vi "Process CAN Frame.vi"(10 "CAN frame":T1 {"type" items=["CAN Data", "CAN Remote"]; "identifier" format="%.0x"}) -> ()   [LabVIEW 2014]
uses:
  <vilib>/RioEmbeddedCAN/RioEmbeddedCAN.llb/CANFrameControl.ctl
  MC/MC Temp 1.ctl
  MC/MC Temp 2.ctl
  MC/MC Temp 3.ctl
  MC/MC Position.ctl
  MC/MC Current.ctl
  MC/MC Voltage.ctl
  MC/MC State.ctl
  Inverter States.ctl
  Inverter Run Modes.ctl
  VSM States.ctl
  MC/MC Faults.ctl
  MC/MC Post Faults.ctl
  MC/MC Run Faults.ctl
  MC/MC Torque.ctl
  Global Data.vi
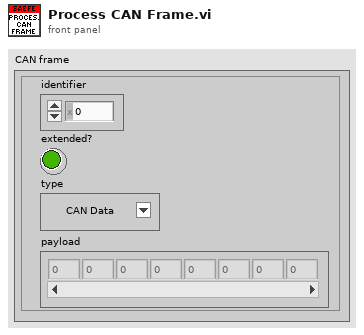
[diagram p1: front panel]
types:
  T1 = typedef "CANFrameControl.ctl" = cluster{"identifier":u32, "extended?":bool, "type":u8, "payload":u8[]}
  T2 = typedef "MC Temp 1.ctl" = cluster{"IGBT A (C)":dbl, "IGBT B (C)":dbl, "IGBT C (C)":dbl, "Gate Driver (C)":dbl}
  T3 = typedef "MC Temp 2.ctl" = cluster{"Control Board (C)":dbl, "RTD #1":dbl, "RTD #2":dbl, "RTD #3":dbl}
  T4 = typedef "MC Temp 3.ctl" = cluster{"RTD #4":dbl, "RTD #5":dbl, "Motor (C)":dbl, "T-Shudder":dbl}
  T5 = typedef "MC Position.ctl" = cluster{"Motor Angle":dbl, "Motor Speed":dbl, "Electrical Output Freq.":dbl, "Delta Resolver Filt.":dbl}
  T6 = typedef "MC Current.ctl" = cluster{"I-Phase A":dbl, "I-Phase B":dbl, "I-Phase C":dbl, "I-Battery":dbl}
  T7 = typedef "MC Voltage.ctl" = cluster{"V-Phase AB":dbl, "V-Phase BC":dbl, "V-Output":dbl, "V-Battery":dbl}
  T8 = typedef "MC State.ctl" = cluster{"Inverter":T9, "Inv. Run Mode":T10, "Inv. Command":enum16{"CAN Mode", "VSM Mode"}, "Inv. Enable":enum16{"Inverter Disabled", "Inverter Enabled"}, "Inv. Enable Lock":enum16{"Inverter Locked", "Inverter Unlocked"}, "Direction":enum16{"Forward", "Reverse/Stopped"}, "VSM States":T11, "Relay 1":bool, "Relay 2":bool, "Relay 3":bool, "Relay 4":bool}
  T9 = typedef "Inverter States.ctl" = enum16{"Power On", "Stop", "Open Loop", "Closed Loop", "Wait", "Internal", "Idle Run", "Idle Stop", ""}
  T10 = typedef "Inverter Run Modes.ctl" = enum16{"Torque Mode", "Speed Mode"}
  T11 = typedef "VSM States.ctl" = enum16{"VSM Start", "Pre-Charge Init", "Pre-Charge Active", "Pre-Charge Complete", "VSM Wait", "VSM Ready", "Motor Running", "Blink Fault Code", "Shutdown in Process", "Recycle Power"}
  T12 = typedef "MC Faults.ctl" = cluster{"POST":T13, "RUN":T14}
  T13 = typedef "MC Post Faults.ctl" = enum32{"None"}
  T14 = typedef "MC Run Faults.ctl" = enum32{"None"}
  T15 = typedef "MC Torque.ctl" = cluster{"T-Requested (Telem)":dbl, "T-Feedback":dbl}
  T16 = enum16{"Off", "On, Not Charging", "Charging", "Charging Finished", "Charging Error"}
  T17 = enum16{"Disconnected", "Pre-charging", "Main Charging", "Balancing", "Charging Finished OK", "Charging Error"}
  T18 = typedef "BMS Telemetry.ctl" = cluster{"Ignition":bool, "Charger Mains":bool, "Fast Charge":bool, "Simple Charger Enabled":bool, "Car State":enum16{"Off", "On, Not Charging", "Charging", "Charging Finished", "Charging Error"}, "Charging State":enum16{"Disconnected", "Pre-charging", "Main Charging", "Balancing", "Charging Finished OK", "Charging Error"}, "Charging Stage Duration":u16, "Last Charging Error":enum16{"No Error", "Cell Voltage Too Low", "No Comm from Cells so can't start", "Maximum charging stage duration expired", "No Comm from Cels so can't balande", "Cannot set balancing voltage", "Cell temps too high", "No Comms so can't determine temp", "# of Cells Mismatch", "Cells Overvoltage", "Cell Protection Event occured."}, "Number of Detected Cells":u8, "Under-Voltage":bool, "Over-Voltage":bool, "Overheat":bool, "Leakage":bool, "No Cell Comms":bool, "Low Voltage":bool, "High Temperature":bool, "Min Cell V":dbl, "Max Cell V":dbl, "Mean Cell V":dbl, "Total V":dbl, "Min Cell t":dbl, "Max Cell t":dbl, "Mean Cell t":dbl, "Cell Voltages":cluster{"[0]":dbl, "[1]":dbl, "[2]":dbl, "[3]":dbl, "[4]":dbl, "[5]":dbl, "[6]":dbl, "[7]":dbl, "[8]":dbl, "[9]":dbl, "[10]":dbl, "[11]":dbl, "[12]":dbl, "[13]":dbl, "[14]":dbl, "[15]":dbl, "[16]":dbl, "[17]":dbl, "[18]":dbl, "[19]":dbl, "[20]":dbl, "[21]":dbl, "[22]":dbl, "[23]":dbl, "[24]":dbl, "[25]":dbl, "[26]":dbl, "[27]":dbl, "[28]":dbl, "[29]":dbl, "[30]":dbl, "[31]":dbl, "[32]":dbl, "[33]":dbl, "[34]":dbl, "[35]":dbl, "[36]":dbl, "[37]":dbl, "[38]":dbl, "[39]":dbl, "[40]":dbl, "[41]":dbl, "[42]":dbl, "[43]":dbl, "[44]":dbl, "[45]":dbl, "[46]":dbl, "[47]":dbl, "[48]":dbl, "[49]":dbl, "[50]":dbl, "[51]":dbl, "[52]":dbl, "[53]":dbl, "[54]":dbl, "[55]":dbl, "[56]":dbl, "[57]":dbl, "[58]":dbl, "[59]":dbl, "[60]":dbl, "[61]":dbl, "[62]":dbl, "[63]":dbl, "[64]":dbl, "[65]":dbl, "[66]":dbl, "[67]":dbl, "[68]":dbl, "[69]":dbl, "[70]":dbl}, "Cell Temps":cluster{"[0]":dbl, "[1]":dbl, "[2]":dbl, "[3]":dbl, "[4]":dbl, "[5]":dbl, "[6]":dbl, "[7]":dbl, "[8]":dbl, "[9]":dbl, "[10]":dbl, "[11]":dbl, "[12]":dbl, "[13]":dbl, "[14]":dbl, "[15]":dbl, "[16]":dbl, "[17]":dbl, "[18]":dbl, "[19]":dbl, "[20]":dbl, "[21]":dbl, "[22]":dbl, "[23]":dbl, "[24]":dbl, "[25]":dbl, "[26]":dbl, "[27]":dbl, "[28]":dbl, "[29]":dbl, "[30]":dbl, "[31]":dbl, "[32]":dbl, "[33]":dbl, "[34]":dbl, "[35]":dbl, "[36]":dbl, "[37]":dbl, "[38]":dbl, "[39]":dbl, "[40]":dbl, "[41]":dbl, "[42]":dbl, "[43]":dbl, "[44]":dbl, "[45]":dbl, "[46]":dbl, "[47]":dbl, "[48]":dbl, "[49]":dbl, "[50]":dbl, "[51]":dbl, "[52]":dbl, "[53]":dbl, "[54]":dbl, "[55]":dbl, "[56]":dbl, "[57]":dbl, "[58]":dbl, "[59]":dbl, "[60]":dbl, "[61]":dbl, "[62]":dbl, "[63]":dbl, "[64]":dbl, "[65]":dbl, "[66]":dbl, "[67]":dbl, "[68]":dbl, "[69]":dbl, "[70]":dbl}}
  T19 = cluster{"[0]":dbl, "[1]":dbl, "[2]":dbl, "[3]":dbl, "[4]":dbl, "[5]":dbl, "[6]":dbl, "[7]":dbl, "[8]":dbl, "[9]":dbl, "[10]":dbl, "[11]":dbl, "[12]":dbl, "[13]":dbl, "[14]":dbl, "[15]":dbl, "[16]":dbl, "[17]":dbl, "[18]":dbl, "[19]":dbl, "[20]":dbl, "[21]":dbl, "[22]":dbl, "[23]":dbl, "[24]":dbl, "[25]":dbl, "[26]":dbl, "[27]":dbl, "[28]":dbl, "[29]":dbl, "[30]":dbl, "[31]":dbl, "[32]":dbl, "[33]":dbl, "[34]":dbl, "[35]":dbl, "[36]":dbl, "[37]":dbl, "[38]":dbl, "[39]":dbl, "[40]":dbl, "[41]":dbl, "[42]":dbl, "[43]":dbl, "[44]":dbl, "[45]":dbl, "[46]":dbl, "[47]":dbl, "[48]":dbl, "[49]":dbl, "[50]":dbl, "[51]":dbl, "[52]":dbl, "[53]":dbl, "[54]":dbl, "[55]":dbl, "[56]":dbl, "[57]":dbl, "[58]":dbl, "[59]":dbl, "[60]":dbl, "[61]":dbl, "[62]":dbl, "[63]":dbl, "[64]":dbl, "[65]":dbl, "[66]":dbl, "[67]":dbl, "[68]":dbl, "[69]":dbl, "[70]":dbl}
  T20 = cluster{"Cell Voltages[0]":dbl, "Cell Voltages[1]":dbl, "Cell Voltages[2]":dbl, "Cell Voltages[3]":dbl, "Cell Voltages[4]":dbl, "Cell Voltages[5]":dbl, "Cell Voltages[6]":dbl, "Cell Voltages[7]":dbl, "Cell Voltages[8]":dbl, "Cell Voltages[9]":dbl, "Cell Voltages[10]":dbl, "Cell Voltages[11]":dbl, "Cell Voltages[12]":dbl, "Cell Voltages[13]":dbl, "Cell Voltages[14]":dbl, "Cell Voltages[15]":dbl, "Cell Voltages[16]":dbl, "Cell Voltages[17]":dbl, "Cell Voltages[18]":dbl, "Cell Voltages[19]":dbl, "Cell Voltages[20]":dbl, "Cell Voltages[21]":dbl, "Cell Voltages[22]":dbl, "Cell Voltages[23]":dbl, "Cell Voltages[24]":dbl, "Cell Voltages[25]":dbl, "Cell Voltages[26]":dbl, "Cell Voltages[27]":dbl, "Cell Voltages[28]":dbl, "Cell Voltages[29]":dbl, "Cell Voltages[30]":dbl, "Cell Voltages[31]":dbl, "Cell Voltages[32]":dbl, "Cell Voltages[33]":dbl, "Cell Voltages[34]":dbl, "Cell Voltages[35]":dbl, "Cell Voltages[36]":dbl, "Cell Voltages[37]":dbl, "Cell Voltages[38]":dbl, "Cell Voltages[39]":dbl, "Cell Voltages[40]":dbl, "Cell Voltages[41]":dbl, "Cell Voltages[42]":dbl, "Cell Voltages[43]":dbl, "Cell Voltages[44]":dbl, "Cell Voltages[45]":dbl, "Cell Voltages[46]":dbl, "Cell Voltages[47]":dbl, "Cell Voltages[48]":dbl, "Cell Voltages[49]":dbl, "Cell Voltages[50]":dbl, "Cell Voltages[51]":dbl, "Cell Voltages[52]":dbl, "Cell Voltages[53]":dbl, "Cell Voltages[54]":dbl, "Cell Voltages[55]":dbl, "Cell Voltages[56]":dbl, "Cell Voltages[57]":dbl, "Cell Voltages[58]":dbl, "Cell Voltages[59]":dbl, "Cell Voltages[60]":dbl, "Cell Voltages[61]":dbl, "Cell Voltages[62]":dbl, "Cell Voltages[63]":dbl, "Cell Voltages[64]":dbl, "Cell Voltages[65]":dbl, "Cell Voltages[66]":dbl, "Cell Voltages[67]":dbl, "Cell Voltages[68]":dbl, "Cell Voltages[69]":dbl, "Cell Voltages[70]":dbl}
  T21 = cluster{"Cell Temps[0]":dbl, "Cell Temps[1]":dbl, "Cell Temps[2]":dbl, "Cell Temps[3]":dbl, "Cell Temps[4]":dbl, "Cell Temps[5]":dbl, "Cell Temps[6]":dbl, "Cell Temps[7]":dbl, "Cell Temps[8]":dbl, "Cell Temps[9]":dbl, "Cell Temps[10]":dbl, "Cell Temps[11]":dbl, "Cell Temps[12]":dbl, "Cell Temps[13]":dbl, "Cell Temps[14]":dbl, "Cell Temps[15]":dbl, "Cell Temps[16]":dbl, "Cell Temps[17]":dbl, "Cell Temps[18]":dbl, "Cell Temps[19]":dbl, "Cell Temps[20]":dbl, "Cell Temps[21]":dbl, "Cell Temps[22]":dbl, "Cell Temps[23]":dbl, "Cell Temps[24]":dbl, "Cell Temps[25]":dbl, "Cell Temps[26]":dbl, "Cell Temps[27]":dbl, "Cell Temps[28]":dbl, "Cell Temps[29]":dbl, "Cell Temps[30]":dbl, "Cell Temps[31]":dbl, "Cell Temps[32]":dbl, "Cell Temps[33]":dbl, "Cell Temps[34]":dbl, "Cell Temps[35]":dbl, "Cell Temps[36]":dbl, "Cell Temps[37]":dbl, "Cell Temps[38]":dbl, "Cell Temps[39]":dbl, "Cell Temps[40]":dbl, "Cell Temps[41]":dbl, "Cell Temps[42]":dbl, "Cell Temps[43]":dbl, "Cell Temps[44]":dbl, "Cell Temps[45]":dbl, "Cell Temps[46]":dbl, "Cell Temps[47]":dbl, "Cell Temps[48]":dbl, "Cell Temps[49]":dbl, "Cell Temps[50]":dbl, "Cell Temps[51]":dbl, "Cell Temps[52]":dbl, "Cell Temps[53]":dbl, "Cell Temps[54]":dbl, "Cell Temps[55]":dbl, "Cell Temps[56]":dbl, "Cell Temps[57]":dbl, "Cell Temps[58]":dbl, "Cell Temps[59]":dbl, "Cell Temps[60]":dbl, "Cell Temps[61]":dbl, "Cell Temps[62]":dbl, "Cell Temps[63]":dbl, "Cell Temps[64]":dbl, "Cell Temps[65]":dbl, "Cell Temps[66]":dbl, "Cell Temps[67]":dbl, "Cell Temps[68]":dbl, "Cell Temps[69]":dbl, "Cell Temps[70]":dbl}
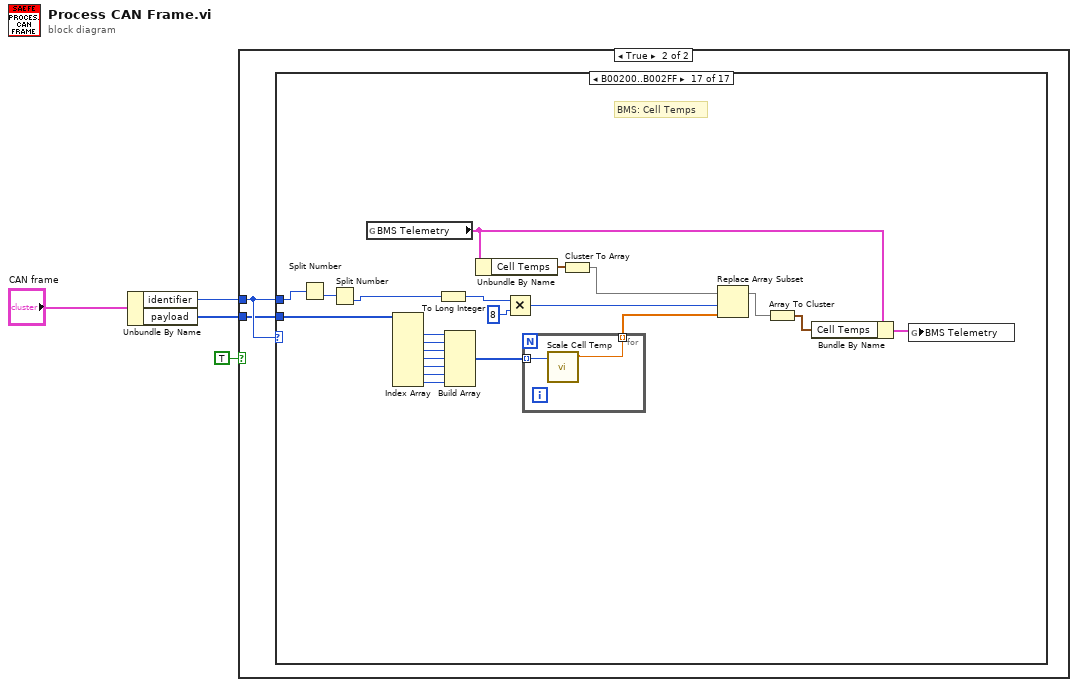
[diagram p0: block diagram]
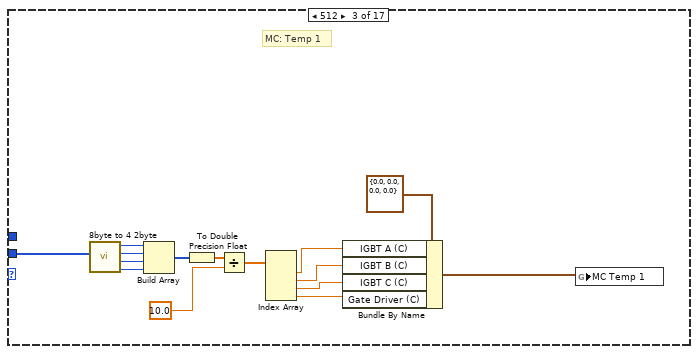
[diagram p5: hidden frame]
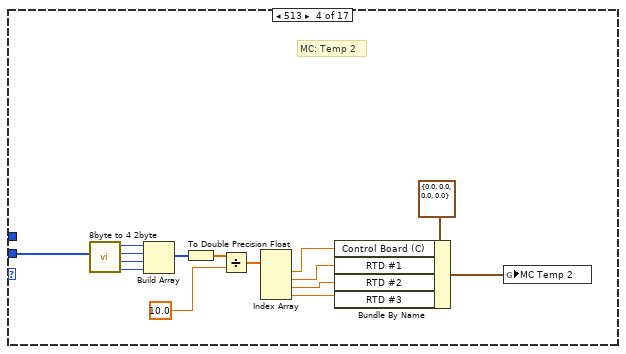
[diagram p6: hidden frame]
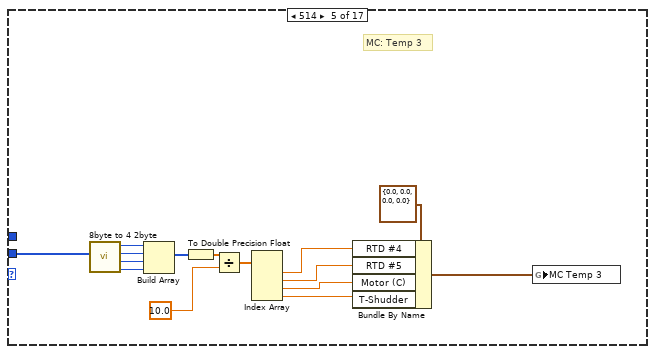
[diagram p7: hidden frame]
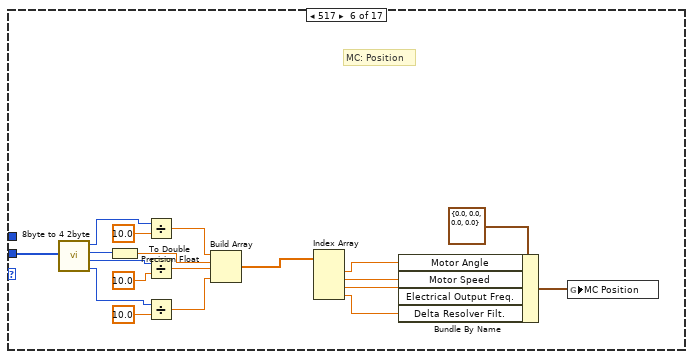
[diagram p8: hidden frame]
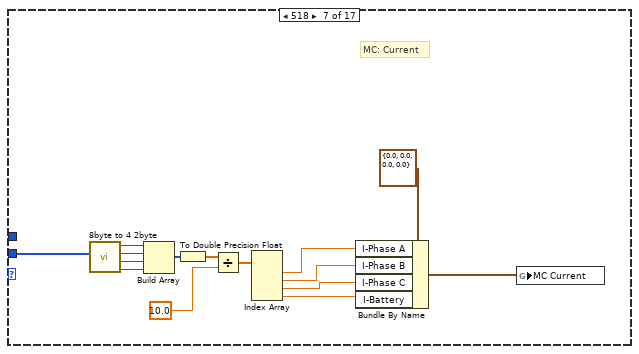
[diagram p9: hidden frame]
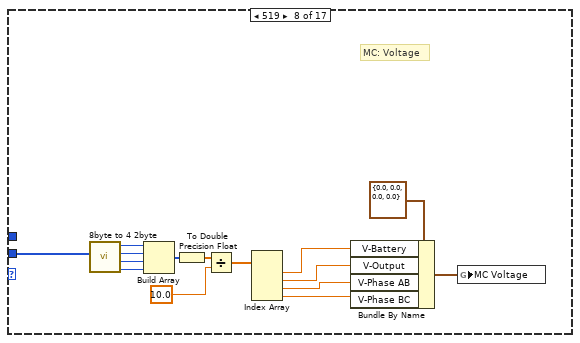
[diagram p10: hidden frame]
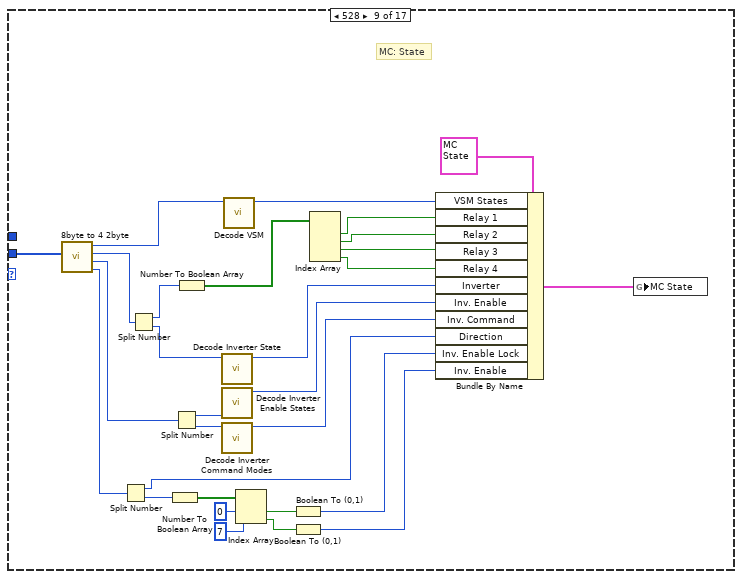
[diagram p11: hidden frame]
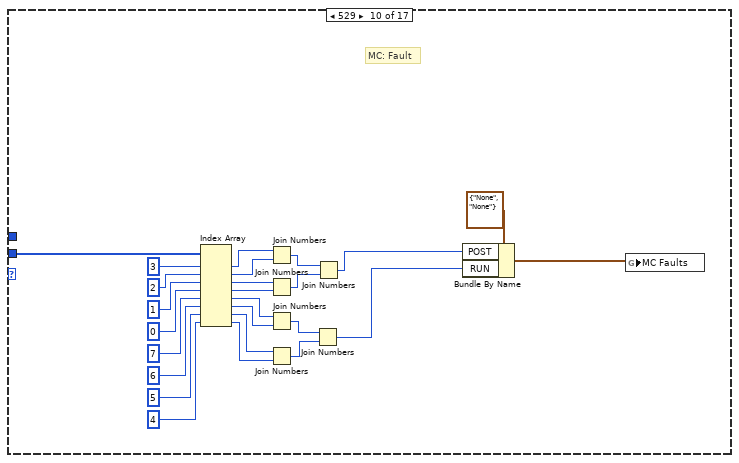
[diagram p12: hidden frame]
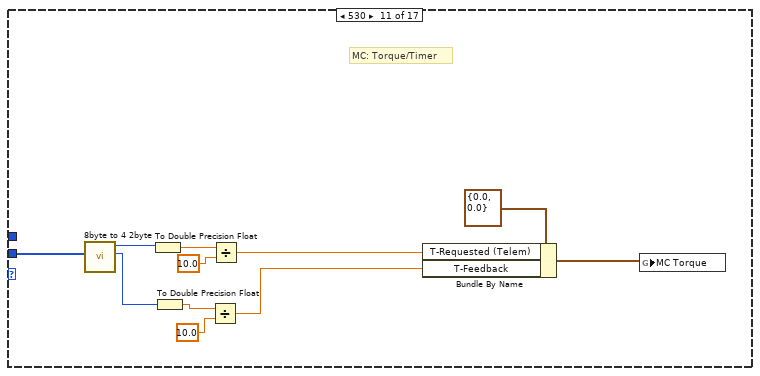
[diagram p13: hidden frame]
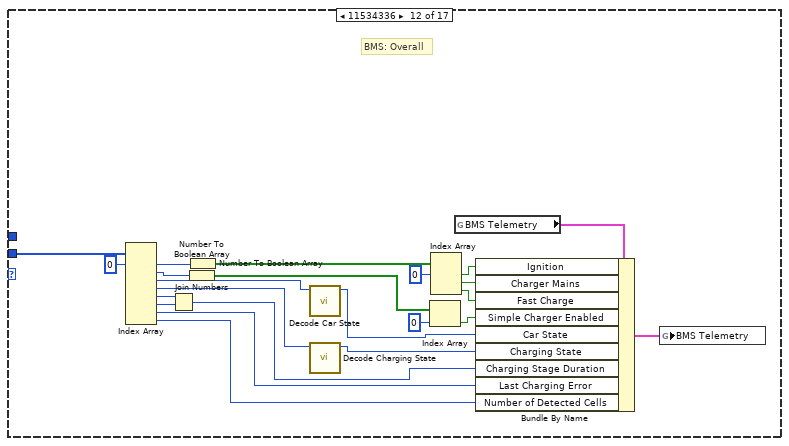
[diagram p14: hidden frame]
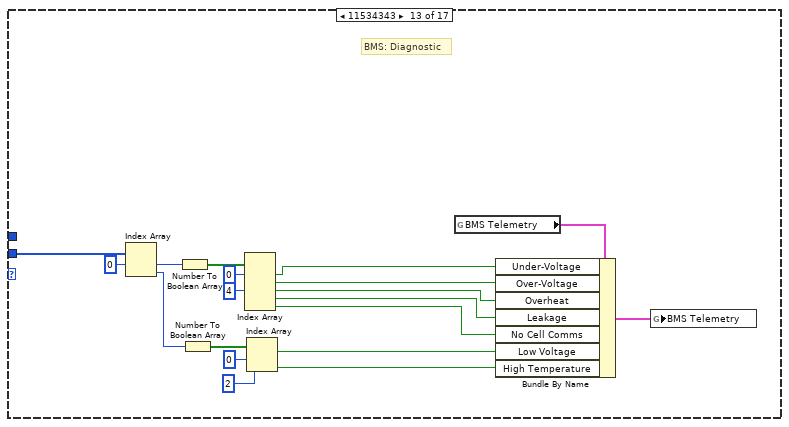
[diagram p15: hidden frame]
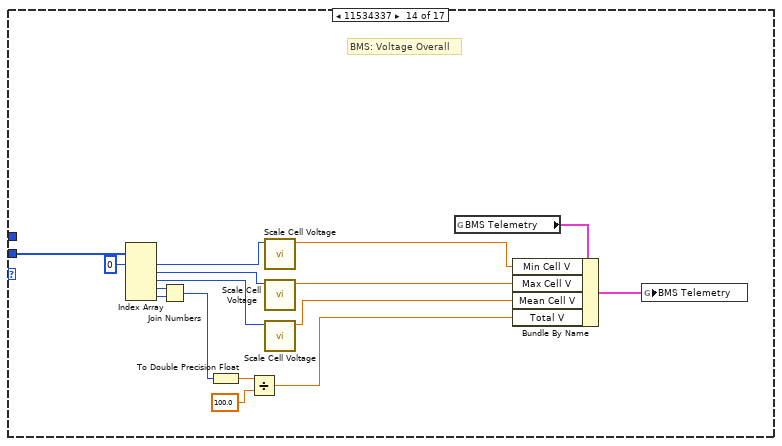
[diagram p16: hidden frame]
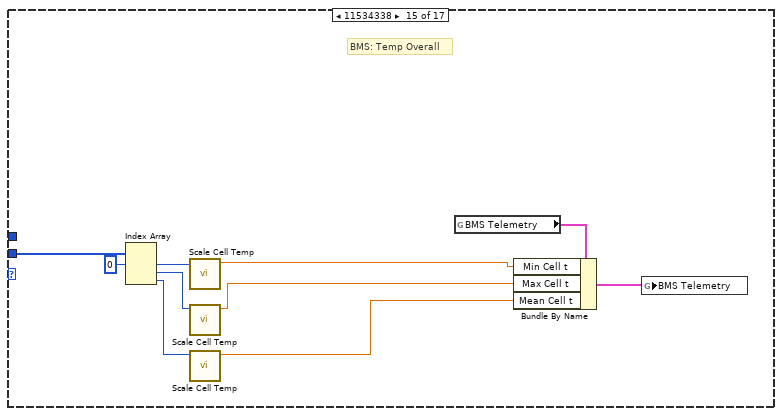
[diagram p17: hidden frame]
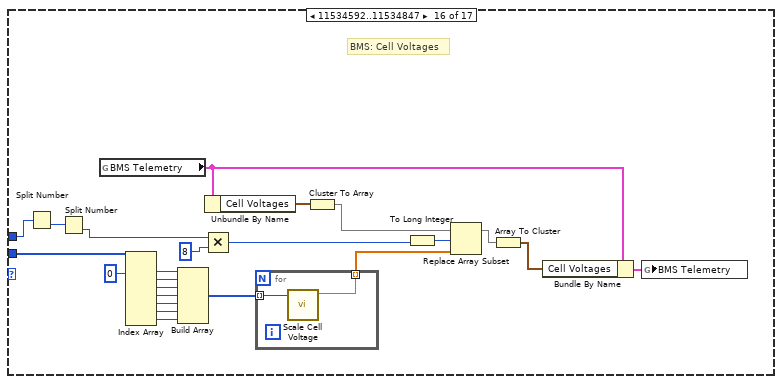
[diagram p18: hidden frame]
diagram:
  n1 = Unbundle By Name("CAN frame") -> ("identifier"=w3:u32, "payload"=w2:u8[])
  n2 = case shown="True" TRUE {
    tunnel: w3 -> [_ w6]
    tunnel: w2 -> [_ w5]
    frame False {
    }
    frame True {
      n3 = case shown="B00200..B002FF" w6 {
        tunnel: w6 -> [_ _ _ _ _ _ _ _ _ _ _ _ _ _ _ w238 w261]
        tunnel: w5 -> [_ _ w21 w36 w51 w70 w85 w100 w103 w132 w165 w166 w189 w221 w231 w251 w274]
        frame 238 {
          # "Unknown CAN Frame"
        }
        frame 0, Default {
          # "Do nothing for NULL frame"
        }
        frame 512 {
          # "MC: Temp 1"
          n4 = call "8byte to 4 2byte.vi"("payload"=w21) -> ("7,6"=w17:i16, "5,4"=w18:i16, "3,2"=w19:i16, "1,0"=w20:i16)  [unwired: 7 in]
          n5 = Build Array(w20, w19, w18, w17) -> (w10:i16[])
          n6 = To Double Precision Float(number=w10) -> (double precision float=w11:dbl[])
          n7 = Divide(x=w11, y=10.0) -> (x/y=w9:dbl[])
          n8 = Index Array(array=w9) -> (element #1=w15:dbl, element #2=w14:dbl, element #3=w13:dbl, element #4=w12:dbl)  [unwired: 4 in]
          n9 = Bundle By Name(cluster=T2 {"IGBT A (C)"=0.0, "IGBT B (C)"=0.0, "IGBT C (C)"=0.0, "Gate Driver (C)"=0.0} ("MC Temp 1"), "IGBT A (C)"=w15, "IGBT B (C)"=w14, "IGBT C (C)"=w13, "Gate Driver (C)"=w12) -> (w7:T2)
          n10 = global write "Global Data.vi" "MC Temp 1"(w7) -> ()
        }
        frame 513 {
          # "MC: Temp 2"
          n11 = call "8byte to 4 2byte.vi"("payload"=w36) -> ("7,6"=w32:i16, "5,4"=w33:i16, "3,2"=w34:i16, "1,0"=w35:i16)  [unwired: 7 in]
          n12 = Build Array(w35, w34, w33, w32) -> (w25:i16[])
          n13 = To Double Precision Float(number=w25) -> (double precision float=w26:dbl[])
          n14 = Divide(x=w26, y=10.0) -> (x/y=w24:dbl[])
          n15 = Index Array(array=w24) -> (element #1=w30:dbl, element #2=w29:dbl, element #3=w28:dbl, element #4=w27:dbl)  [unwired: 4 in]
          n16 = Bundle By Name(cluster=T3 {"Control Board (C)"=0.0, "RTD #1"=0.0, "RTD #2"=0.0, "RTD #3"=0.0} ("MC Temp 2"), "Control Board (C)"=w30, "RTD #1"=w29, "RTD #2"=w28, "RTD #3"=w27) -> (w23:T3)
          n17 = global write "Global Data.vi" "MC Temp 2"(w23) -> ()
        }
        frame 514 {
          # "MC: Temp 3"
          n18 = call "8byte to 4 2byte.vi"("payload"=w51) -> ("7,6"=w47:i16, "5,4"=w48:i16, "3,2"=w49:i16, "1,0"=w50:i16)  [unwired: 7 in]
          n19 = Build Array(w50, w49, w48, w47) -> (w40:i16[])
          n20 = To Double Precision Float(number=w40) -> (double precision float=w41:dbl[])
          n21 = Divide(x=w41, y=10.0) -> (x/y=w39:dbl[])
          n22 = Index Array(array=w39) -> (element #1=w45:dbl, element #2=w44:dbl, element #3=w43:dbl, element #4=w42:dbl)  [unwired: 4 in]
          n23 = Bundle By Name(cluster=T4 {"RTD #4"=0.0, "RTD #5"=0.0, "Motor (C)"=0.0, "T-Shudder"=0.0} ("MC Temp 3"), "RTD #4"=w45, "RTD #5"=w44, "Motor (C)"=w43, "T-Shudder"=w42) -> (w38:T4)
          n24 = global write "Global Data.vi" "MC Temp 3"(w38) -> ()
        }
        frame 517 {
          # "MC: Position"
          n25 = call "8byte to 4 2byte.vi"("payload"=w70) -> ("7,6"=w65:i16, "5,4"=w66:i16, "3,2"=w60:i16, "1,0"=w69:i16)  [unwired: 7 in]
          n26 = To Double Precision Float(number=w60) -> (double precision float=w59:dbl)
          n27 = Divide(x=w69, y=10.0) -> (x/y=w64:dbl)
          n28 = Divide(x=w66, y=10.0) -> (x/y=w63:dbl)
          n29 = Divide(x=w65, y=10.0) -> (x/y=w62:dbl)
          n30 = Build Array(w64, w59, w63, w62) -> (w58:dbl[])
          n31 = Index Array(array=w58) -> (element #1=w57:dbl, element #2=w56:dbl, element #3=w55:dbl, element #4=w54:dbl)  [unwired: 4 in]
          n32 = Bundle By Name(cluster=T5 {"Motor Angle"=0.0, "Motor Speed"=0.0, "Electrical Output Freq."=0.0, "Delta Resolver Filt."=0.0} ("MC Position"), "Motor Angle"=w57, "Motor Speed"=w56, "Electrical Output Freq."=w55, "Delta Resolver Filt."=w54) -> (w52:T5)
          n33 = global write "Global Data.vi" "MC Position"(w52) -> ()
        }
        frame 518 {
          # "MC: Current"
          n34 = call "8byte to 4 2byte.vi"("payload"=w85) -> ("7,6"=w81:i16, "5,4"=w82:i16, "3,2"=w83:i16, "1,0"=w84:i16)  [unwired: 7 in]
          n35 = Build Array(w84, w83, w82, w81) -> (w74:i16[])
          n36 = To Double Precision Float(number=w74) -> (double precision float=w75:dbl[])
          n37 = Divide(x=w75, y=10.0) -> (x/y=w73:dbl[])
          n38 = Index Array(array=w73) -> (element #1=w79:dbl, element #2=w78:dbl, element #3=w77:dbl, element #4=w76:dbl)  [unwired: 4 in]
          n39 = Bundle By Name(cluster=T6 {"I-Phase A"=0.0, "I-Phase B"=0.0, "I-Phase C"=0.0, "I-Battery"=0.0} ("MC Current"), "I-Phase A"=w79, "I-Phase B"=w78, "I-Phase C"=w77, "I-Battery"=w76) -> (w71:T6)
          n40 = global write "Global Data.vi" "MC Current"(w71) -> ()
        }
        frame 519 {
          # "MC: Voltage"
          n41 = call "8byte to 4 2byte.vi"("payload"=w100) -> ("7,6"=w96:i16, "5,4"=w97:i16, "3,2"=w98:i16, "1,0"=w99:i16)  [unwired: 7 in]
          n42 = Build Array(w99, w98, w97, w96) -> (w90:i16[])
          n43 = To Double Precision Float(number=w90) -> (double precision float=w91:dbl[])
          n44 = Divide(x=w91, y=10.0) -> (x/y=w89:dbl[])
          n45 = Index Array(array=w89) -> (element #1=w95:dbl, element #2=w94:dbl, element #3=w93:dbl, element #4=w92:dbl)  [unwired: 4 in]
          n46 = Bundle By Name(cluster=T7 {"V-Phase AB"=0.0, "V-Phase BC"=0.0, "V-Output"=0.0, "V-Battery"=0.0} ("MC Voltage"), "V-Battery"=w95, "V-Output"=w94, "V-Phase AB"=w93, "V-Phase BC"=w92) -> (w87:T7)
          n47 = global write "Global Data.vi" "MC Voltage"(w87) -> ()
        }
        frame 528 {
          # "MC: State"
          n48 = call "8byte to 4 2byte.vi"("payload"=w103) -> ("7,6"=w112:i16, "5,4"=w125:i16, "3,2"=w128:i16, "1,0"=w129:i16)  [unwired: 7 in]
          n49 = Split Number(x=w112) -> (hi(x)=w111:u8, lo(x)=w120:u8)
          n50 = Split Number(x=w128) -> (hi(x)=w104:u8, lo(x)=w127:u8)
          n51 = Number To Boolean Array(number=w120) -> (Boolean array=w119:bool[])
          n52 = Split Number(x=w125) -> (hi(x)=w124:u8, lo(x)=w122:u8)
          n53 = Number To Boolean Array(number=w104) -> (Boolean array=w110:bool[])
          n54 = call "Decode Inverter State.vi"("Byte In"=w127) -> ("Inverter State Out"=w126:T9)  [unwired: 10 in]
          n55 = call "Decode Inverter Enable States.vi"("Numeric"=w124) -> ("Inv. Enable"=w123:enum16{"Inverter Disabled", "Inverter Enabled"})  [unwired: 10 in]
          n56 = call "Decode Inverter Command Modes.vi"("Numeric"=w122) -> ("Inv. Command"=w121:enum16{"CAN Mode", "VSM Mode"})  [unwired: 10 in]
          n57 = call "Decode VSM.vi"("VSM Word"=w129) -> ("Enum"=w105:T11)  [unwired: 10 in]
          n58 = Index Array(array=w119, index #1=0 ("index"), index #2=7 ("index")) -> (element #1=w116:bool, element #2=w114:bool)
          n59 = Boolean To (0,1)(Boolean=w116) -> (0, 1=w115:i16)
          n60 = Boolean To (0,1)(Boolean=w114) -> (0, 1=w113:i16)
          n61 = Index Array(array=w110) -> (element #1=w109:bool, element #2=w108:bool, element #3=w107:bool, element #4=w106:bool)  [unwired: 4 in]
          n62 = Bundle By Name(cluster=T8 {"Inverter"=enum."Power On", "Inv. Run Mode"=enum."Torque Mode", "Inv. Command"=enum."CAN Mode", "Inv. Enable"=enum."Inverter Disabled", "Inv. Enable Lock"=enum."Inverter Locked", "Direction"=enum."Forward", "VSM States"=enum."VSM Start", "Relay 1"=FALSE, "Relay 2"=FALSE, "Relay 3"=FALSE, "Relay 4"=FALSE} ("MC State"), "VSM States"=w105, "Relay 1"=w109, "Relay 2"=w108, "Relay 3"=w107, "Relay 4"=w106, "Inverter"=w126, "Inv. Enable"=w123, "Inv. Command"=w121, "Direction"=w111, "Inv. Enable Lock"=w115, "Inv. Enable"=w113) -> (w101:T8)
          n63 = global write "Global Data.vi" "MC State"(w101) -> ()
        }
        frame 529 {
          # "MC: Fault"
          n64 = Index Array(array=w132, index #1=3 ("index"), index #2=2 ("index"), index #3=1 ("index"), index #4=0 ("index"), index #5=7 ("index"), index #6=6 ("index"), index #7=5 ("index"), index #8=4 ("index")) -> (element #1=w142:u8, element #2=w141:u8, element #3=w140:u8, element #4=w139:u8, element #5=w138:u8, element #6=w137:u8, element #7=w136:u8, element #8=w135:u8)
          n65 = Join Numbers(hi=w142, lo=w141) -> ((hi.lo)=w143:u16)
          n66 = Join Numbers(hi=w140, lo=w139) -> ((hi.lo)=w144:u16)
          n67 = Join Numbers(hi=w138, lo=w137) -> ((hi.lo)=w145:u16)
          n68 = Join Numbers(hi=w136, lo=w135) -> ((hi.lo)=w146:u16)
          n69 = Join Numbers(hi=w145, lo=w146) -> ((hi.lo)=w133:u32)
          n70 = Join Numbers(hi=w143, lo=w144) -> ((hi.lo)=w134:u32)
          n71 = Bundle By Name(cluster=T12 {"POST"=enum."None", "RUN"=enum."None"} ("MC Faults"), "POST"=w134, "RUN"=w133) -> (w130:T12)
          n72 = global write "Global Data.vi" "MC Faults"(w130) -> ()
        }
        frame 530 {
          # "MC: Torque/Timer"
          n73 = call "8byte to 4 2byte.vi"("payload"=w165) -> ("3,2"=w161:i16, "1,0"=w164:i16)  [unwired: 7 in, 2 out]
          n74 = To Double Precision Float(number=w164) -> (double precision float=w163:dbl)
          n75 = To Double Precision Float(number=w161) -> (double precision float=w160:dbl)
          n76 = Divide(x=w160, y=10.0) -> (x/y=w157:dbl)
          n77 = Divide(x=w163, y=10.0) -> (x/y=w158:dbl)
          n78 = Bundle By Name(cluster=T15 {"T-Requested (Telem)"=0.0, "T-Feedback"=0.0} ("MC Torque"), "T-Requested (Telem)"=w158, "T-Feedback"=w157) -> (w156:T15)
          n79 = global write "Global Data.vi" "MC Torque"(w156) -> ()
        }
        frame 11534336 {
          # "BMS: Overall"
          n80 = Index Array(array=w166, index #1=0 ("index")) -> (element #1=w185:u8, element #2=w179:u8, element #3=w174:u8, element #4=w173:u8, element #5=w171:u8, element #6=w170:u8, element #7=w168:u8, element #8=w167:u8)  [unwired: 7 in]
          n81 = Join Numbers(hi=w171, lo=w170) -> ((hi.lo)=w169:u16)
          n82 = Number To Boolean Array(number=w179) -> (Boolean array=w177:bool[])
          n83 = Number To Boolean Array(number=w185) -> (Boolean array=w184:bool[])
          n84 = call "Decode Car State.vi"("Numeric"=w174) -> ("Car State"=w175:T16)  [unwired: 10 in]
          n85 = call "Decode Charging State.vi"("Numeric"=w173) -> ("Charging State"=w172:T17)  [unwired: 10 in]
          n86 = Index Array(array=w177, index=0) -> (element=w178:bool)
          n87 = Index Array(array=w184, index #1=0 ("index")) -> (element #1=w182:bool, element #2=w181:bool, element #3=w180:bool)  [unwired: 2 in]
          n88 = global read "Global Data.vi" "BMS Telemetry"() -> (w188:T18)
          n89 = Bundle By Name(cluster=w188, "Ignition"=w182, "Charger Mains"=w181, "Fast Charge"=w180, "Simple Charger Enabled"=w178, "Car State"=w175, "Charging State"=w172, "Charging Stage Duration"=w169, "Last Charging Error"=w168, "Number of Detected Cells"=w167) -> (w187:T18)
          n90 = global write "Global Data.vi" "BMS Telemetry"(w187) -> ()
        }
        frame 11534343 {
          # "BMS: Diagnostic"
          n91 = Index Array(array=w189, index #1=0 ("index")) -> (element #1=w204:u8, element #2=w195:u8)  [unwired: 1 in]
          n92 = Number To Boolean Array(number=w204) -> (Boolean array=w203:bool[])
          n93 = Number To Boolean Array(number=w195) -> (Boolean array=w194:bool[])
          n94 = Index Array(array=w203, index #1=0 ("index"), index #3=4 ("index")) -> (element #1=w201:bool, element #2=w200:bool, element #3=w198:bool, element #4=w197:bool, element #5=w196:bool)  [unwired: 3 in]
          n95 = Index Array(array=w194, index #1=0 ("index"), index #2=2 ("index")) -> (element #1=w191:bool, element #2=w190:bool)
          n96 = global read "Global Data.vi" "BMS Telemetry"() -> (w207:T18)
          n97 = Bundle By Name(cluster=w207, "Under-Voltage"=w201, "Over-Voltage"=w200, "Overheat"=w198, "Leakage"=w197, "No Cell Comms"=w196, "Low Voltage"=w191, "High Temperature"=w190) -> (w206:T18)
          n98 = global write "Global Data.vi" "BMS Telemetry"(w206) -> ()
        }
        frame 11534337 {
          # "BMS: Voltage Overall"
          n99 = Index Array(array=w221, index #1=0 ("index")) -> (element #1=w219:u8, element #2=w218:u8, element #3=w217:u8, element #4=w216:u8, element #5=w215:u8)  [unwired: 4 in]
          n100 = Join Numbers(hi=w216, lo=w215) -> ((hi.lo)=w214:u16)
          n101 = To Double Precision Float(number=w214) -> (double precision float=w213:dbl)
          n102 = Divide(x=w213, y=100.0) -> (x/y=w208:dbl)
          n103 = call "Scale Cell Voltage.vi"("Numeric in"=w219) -> ("Numeric out"=w211:dbl)  [unwired: 10 in]
          n104 = call "Scale Cell Voltage.vi"("Numeric in"=w218) -> ("Numeric out"=w210:dbl)  [unwired: 10 in]
          n105 = call "Scale Cell Voltage.vi"("Numeric in"=w217) -> ("Numeric out"=w209:dbl)  [unwired: 10 in]
          n106 = global read "Global Data.vi" "BMS Telemetry"() -> (w223:T18)
          n107 = Bundle By Name(cluster=w223, "Min Cell V"=w211, "Max Cell V"=w210, "Mean Cell V"=w209, "Total V"=w208) -> (w222:T18)
          n108 = global write "Global Data.vi" "BMS Telemetry"(w222) -> ()
        }
        frame 11534338 {
          # "BMS: Temp Overall"
          n109 = Index Array(array=w231, index #1=0 ("index")) -> (element #1=w229:u8, element #2=w228:u8, element #3=w227:u8)  [unwired: 2 in]
          n110 = call "Scale Cell Temp.vi"("Numeric in"=w229) -> ("Numeric out"=w226:dbl)  [unwired: 10 in]
          n111 = call "Scale Cell Temp.vi"("Numeric in"=w228) -> ("Numeric out"=w225:dbl)  [unwired: 10 in]
          n112 = call "Scale Cell Temp.vi"("Numeric in"=w227) -> ("Numeric out"=w224:dbl)  [unwired: 10 in]
          n113 = global read "Global Data.vi" "BMS Telemetry"() -> (w233:T18)
          n114 = Bundle By Name(cluster=w233, "Min Cell t"=w226, "Max Cell t"=w225, "Mean Cell t"=w224) -> (w232:T18)
          n115 = global write "Global Data.vi" "BMS Telemetry"(w232) -> ()
        }
        frame 11534592..11534847 {
          # "BMS: Cell Voltages"
          n116 = Split Number(x=w238) -> (lo(x)=w237:u16)  [unwired: 1 out]
          n117 = Split Number(x=w237) -> (lo(x)=w236:u8)  [unwired: 1 out]
          n118 = global read "Global Data.vi" "BMS Telemetry"() -> (w254:T18)
          n119 = Index Array(array=w251, index #1=0 ("index")) -> (element #1=w246:u8, element #2=w245:u8, element #3=w244:u8, element #4=w243:u8, element #5=w242:u8, element #6=w241:u8, element #7=w240:u8)  [unwired: 6 in]
          n120 = Build Array(w246, w245, w244, w243, w242, w241, w240) -> (w253:u8[])
          n121 = Multiply(x=w236, y=u8 8) -> (x*y=w234:u8)
          n122 = Unbundle By Name(w254) -> ("Cell Voltages"=w250:T19)
          n123 = for {
            tunnel: w253 -> [w257] mode=indexing
            tunnel: [w258] -> w252 mode=indexing
            n124 = call "Scale Cell Voltage.vi"("Numeric in"=w257) -> ("Numeric out"=w258:dbl)  [unwired: 10 in]
          }
          n125 = Cluster To Array(cluster=w250) -> (array=w249:dbl[])
          n126 = To Long Integer(number=w234) -> (32bit integer=w235:i32)
          n127 = Replace Array Subset(array=w249, new element=w252, index=w235) -> (w248:dbl[])
          n128 = Array To Cluster(array=w248) -> (cluster=w247:T20)
          n129 = Bundle By Name(cluster=w254, "Cell Voltages"=w247) -> (w256:T18)
          n130 = global write "Global Data.vi" "BMS Telemetry"(w256) -> ()
        }
        frame 11534848..11535103 {
          # "BMS: Cell Temps"
          n131 = Split Number(x=w261) -> (lo(x)=w260:u16)  [unwired: 1 out]
          n132 = Split Number(x=w260) -> (lo(x)=w259:u8)  [unwired: 1 out]
          n133 = global read "Global Data.vi" "BMS Telemetry"() -> (w278:T18)
          n134 = Index Array(array=w274) -> (element #1=w268:u8, element #2=w267:u8, element #3=w266:u8, element #4=w265:u8, element #5=w264:u8, element #6=w263:u8, element #7=w262:u8)  [unwired: 7 in]
          n135 = To Long Integer(number=w259) -> (32bit integer=w273:i32)
          n136 = Build Array(w268, w267, w266, w265, w264, w263, w262) -> (w277:u8[])
          n137 = Unbundle By Name(w278) -> ("Cell Temps"=w272:T19)
          n138 = Multiply(x=w273, y=8) -> (x*y=w275:i32)
          n139 = for {
            tunnel: w277 -> [w281] mode=indexing
            tunnel: [w282] -> w276 mode=indexing
            n140 = call "Scale Cell Temp.vi"("Numeric in"=w281) -> ("Numeric out"=w282:dbl)  [unwired: 10 in]
          }
          n141 = Cluster To Array(cluster=w272) -> (array=w271:dbl[])
          n142 = Replace Array Subset(array=w271, new element=w276, index=w275) -> (w270:dbl[])
          n143 = Array To Cluster(array=w270) -> (cluster=w269:T21)
          n144 = Bundle By Name(cluster=w278, "Cell Temps"=w269) -> (w280:T18)
          n145 = global write "Global Data.vi" "BMS Telemetry"(w280) -> ()
        }
      }
    }
  }
